vi "Write task.vi"(8 "error in (no error)":errorcluster, 10 "task":refnum<k21>, 11 "CompactDAQ in":refnum<class "CompactDAQ.lvclass">) -> (0 "error out":errorcluster, 3 "CompactDAQ out":refnum<class "CompactDAQ.lvclass">)   [LabVIEW 2016, in "CompactDAQ.lvclass"]
uses:
  CompactDAQ.lvclass
  CompactDAQ.lvclass/CompactDAQ.ctl
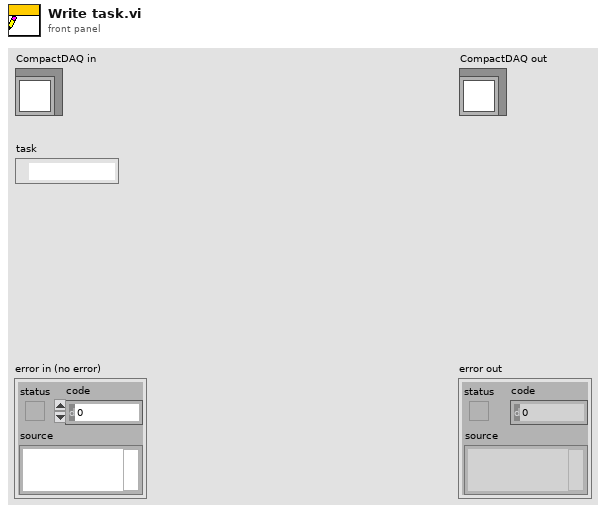
[diagram p1: front panel]
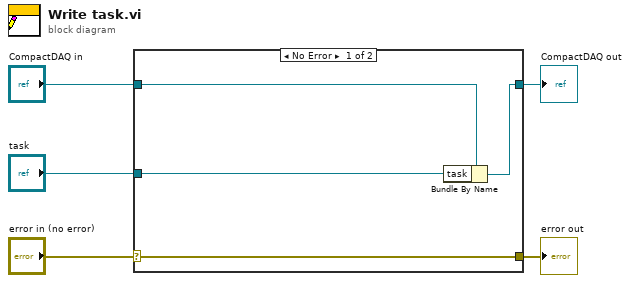
[diagram p0: block diagram]
diagram:
  n1 = case shown="No Error" "error in (no error)" {
    selector: "error in (no error)" -> [w9 w10]
    tunnel: [w9 w10] -> w4
    tunnel: [w7 w11] -> w2
    tunnel: "CompactDAQ in" -> [w8 w11]
    tunnel: "task" -> [w6 _]
    frame No Error {
      n2 = Bundle By Name(cluster=w8, "task"=w6) -> (w7:refnum<class "CompactDAQ.lvclass">)
    }
    frame Error {
    }
  }
  "error out" <- w4
  "CompactDAQ out" <- w2
